vi "Device Init.vi"(0 "IP Address":string="192.168.1.99", 1 "Bytes to Read":u32=52, 5 "Port":string="3000", 11 "Error In":errorcluster) -> (3 "Connected?":bool, 4 "VISA resource name":refnum<visa-resource-name>, 6 "Device":string, 8 "Serial Number":string, 15 "Error Out":errorcluster)   [LabVIEW 2025]
uses:
  <vilib>/Instr/_visa.llb/VISA Open Access Mode.ctl
panel:
  in  "Access Mode":T1 items=["VISA Defaults"=0, "Exclusive Lock"=1, "Load Configured Settings"=4]
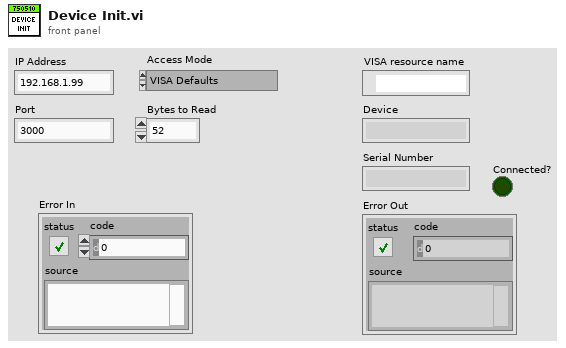
[diagram p1: front panel]
types:
  T1 = typedef "VISA Open Access Mode.ctl" = u32
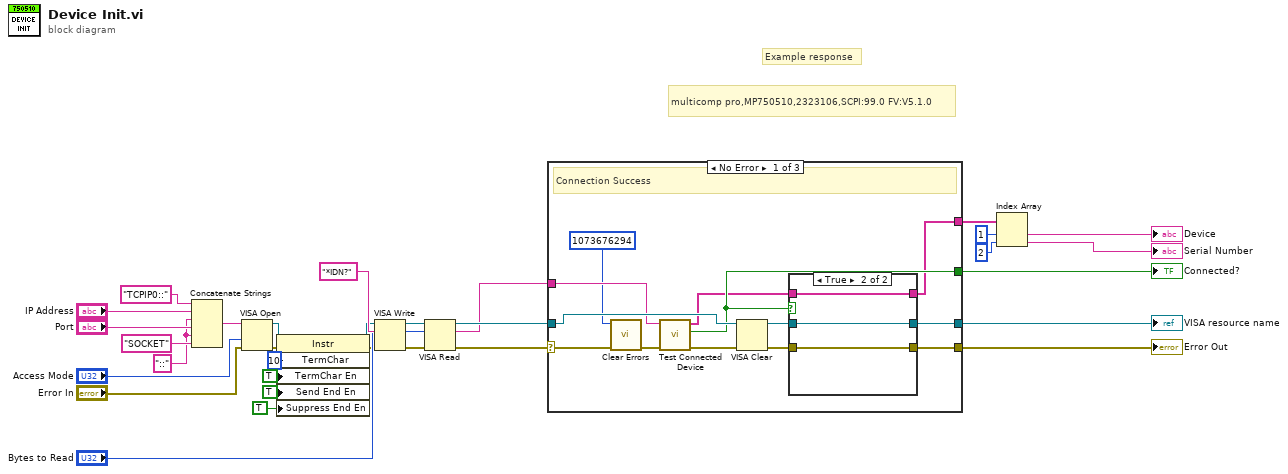
[diagram p0: block diagram]
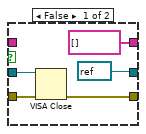
[diagram p2: hidden frame]
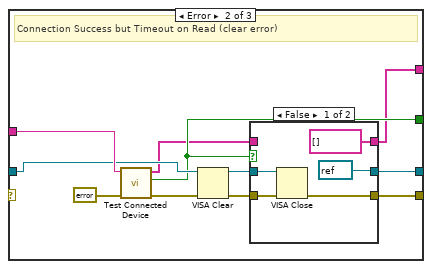
[diagram p3: hidden frame]
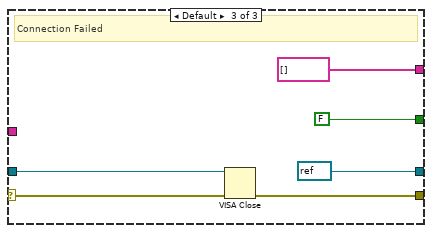
[diagram p5: hidden frame]
diagram:
  w23 = "::"
  # "Example response"
  # "multicomp pro,MP750510,2323106,SCPI:99.0 FV:V5.1.0"
  n1 = Concatenate Strings("TCPIP0::", "IP Address", w23, "Port", w23, "SOCKET") -> (w10:string)
  n2 = VISA Open(access mode="Access Mode", error in (no error)="Error In", VISA resource name=w10) -> (VISA resource name=w5:refnum<visa-resource-name>, error out=w6:errorcluster)  [unwired: 2 in]
  n3 = property class="Instr"(reference=w5, error in=w6, "TermChar"=u8 10 ("Message Based Settings:Termination Character"), "TermChar En"=TRUE ("Message Based Settings:Termination Character Enable"), "Send End En"=TRUE ("Message Based Settings:Send End Enable"), "Suppress End En"=TRUE ("Message Based Settings:Suppress End Enable")) -> (reference out=w4:refnum<visa-resource-name>, error out=w3:errorcluster)
  n4 = VISA Write(VISA resource name=w4, write buffer="*IDN?", error in (no error)=w3) -> (VISA resource name out=w27:refnum<visa-resource-name>, error out=w26:errorcluster)  [unwired: 1 out]
  n5 = VISA Read(VISA resource name=w27, byte count="Bytes to Read", error in (no error)=w26) -> (VISA resource name out=w20:refnum<visa-resource-name>, read buffer=w19:string, error out=w21:errorcluster)  [unwired: 1 out]
  n6 = case shown="No Error" w21 {
    selector: w21 -> [w37 _ w76]
    tunnel: w20 -> [w41 w62 w74]
    tunnel: w19 -> [w35 w63 _]
    tunnel: [w40 w58 w75] -> w17
    tunnel: [w39 w57 refnum<visa-resource-name> refnum ("VISA resource name")] -> w9
    tunnel: [w38 w61 FALSE] -> w18
    tunnel: [w32 w53 string[] [] ("Device Info")] -> w16
    frame No Error {
      # "Connection Success"
      n7 = call <vilib>:"Clear Errors.vi"("error in (no error)"=w37, "specific error code to clear (0: all)"=1073676294) -> ("error out"=w36:errorcluster)  [unwired: 4 in, 1 out]
      n8 = call "Test Connected Device.vi"("error in (no error)"=w36, "Read Buffer"=w35) -> ("error out"=w42:errorcluster, "Connected"=w38:bool, "Device Info"=w33:string[])  [unwired: 7 in]
      n9 = VISA Clear(VISA resource name=w41, error in (no error)=w42) -> (VISA resource name out=w43:refnum<visa-resource-name>, error out=w44:errorcluster)
      n10 = case shown="True" w38 {
        tunnel: [w49 w52] -> w40
        tunnel: w43 -> [w48 w51]
        tunnel: w44 -> [w47 w52]
        tunnel: [refnum<visa-resource-name> refnum ("VISA resource name") w51] -> w39
        tunnel: [string[] [] ("Device Info") w50] -> w32
        tunnel: w33 -> [_ w50]
        frame False {
          n11 = VISA Close(VISA resource name=w48, error in (no error)=w47) -> (error out=w49:errorcluster)
        }
        frame True {
        }
      }
    }
    frame Error {
      # "Connection Success but Timeout on Read (clear error)"
      n12 = call "Test Connected Device.vi"("error in (no error)"=errorcluster {"status"=FALSE, "code"=0, "source"=""} ("error IO"), "Read Buffer"=w63) -> ("error out"=w55:errorcluster, "Connected"=w61:bool, "Device Info"=w54:string[])  [unwired: 7 in]
      n13 = VISA Clear(VISA resource name=w62, error in (no error)=w55) -> (VISA resource name out=w59:refnum<visa-resource-name>, error out=w60:errorcluster)
      n14 = case shown="False" w61 {
        tunnel: [w68 w71] -> w58
        tunnel: w59 -> [w67 w70]
        tunnel: w60 -> [w66 w71]
        tunnel: [refnum<visa-resource-name> refnum ("VISA resource name") w70] -> w57
        tunnel: [string[] [] ("Device Info") w69] -> w53
        tunnel: w54 -> [_ w69]
        frame False {
          n15 = VISA Close(VISA resource name=w67, error in (no error)=w66) -> (error out=w68:errorcluster)
        }
        frame True {
        }
      }
    }
    frame Default {
      # "Connection Failed"
      n16 = VISA Close(VISA resource name=w74, error in (no error)=w76) -> (error out=w75:errorcluster)
    }
  }
  "Error Out" <- w17
  "Connected?" <- w18
  "VISA resource name" <- w9
  n17 = Index Array(array=w16, index #1=1 ("index"), index #2=2 ("index")) -> (element #1=→"Device":string, element #2=→"Serial Number":string)
